vi "Usówanie czasów kas.vi"(10 "Liczba kas":u8, 11 "Czas":timestamp[](array[timestamp])) -> ()   [LabVIEW 2014]
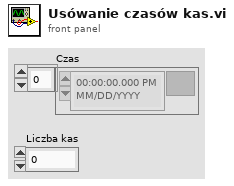
[diagram p1: front panel]
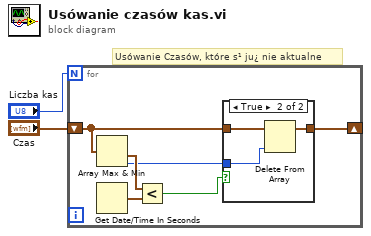
[diagram p0: block diagram]
diagram:
  # "Usówanie Czasów, które s¹ ju¿ nie aktualne"
  n1 = for {
    N: "Liczba kas" -> [_]
    shift-right: [w3] -> _
    shift-left: "Czas" -> [w5]
    n2 = Array Max & Min(array=w5) -> (min value=w7:timestamp, min index (indices)=w4:i32)  [unwired: 2 out]
    n3 = Get Date/Time In Seconds() -> (seconds since 1Jan1904=w8:timestamp)
    n4 = Less?(x=w7, y=w8) -> (x < y?=w6:bool)
    n5 = case shown="True" w6 {
      tunnel: w5 -> [w9 w12]
      tunnel: w4 -> [_ w11]
      tunnel: [w9 w10] -> w3
      frame False {
      }
      frame True {
        n6 = Delete From Array(array=w12, index=w11) -> (array with subset deleted=w10:timestamp[])  [unwired: 1 in, 1 out]
      }
    }
  }
